vi "updateCVTCluster.vi"(1 "error in":errorcluster, 2 "variant (destination) out":variant, 3 "Cluster Names":string[](array[string]), 4 "CVT Names":string[](array[string])) -> (0 "error out":errorcluster)   [LabVIEW 2011]
uses:
  OnOffTypeDef.ctl
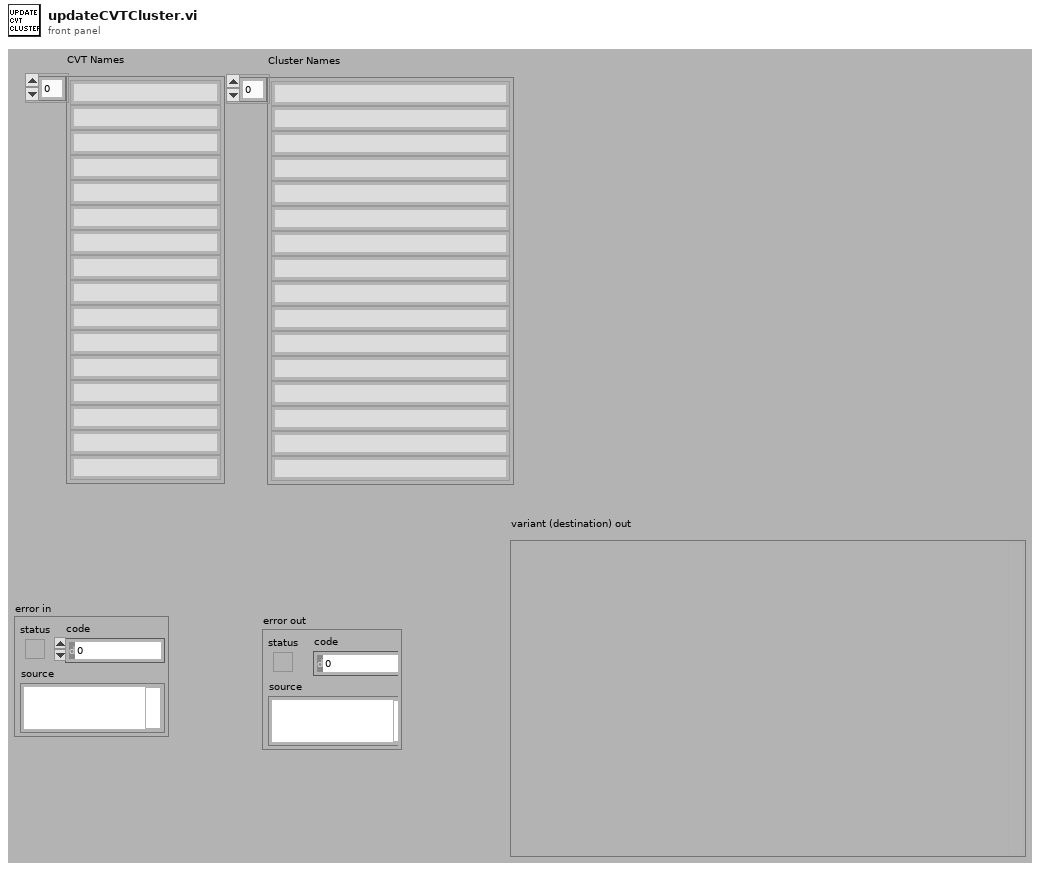
[diagram p1: front panel]
types:
  T1 = typedef "OnOffTypeDef.ctl" = enum16{"off", "on"}
  T2 = typedef "Type Descriptor Enumeration__ogtk.ctl" = enum8{"<Null>", "I8", "I16", "I32", "I64", "U8", "U16", "U32", "U64", "SGL", "DBL", "EXT", "CSG", "CDB", "CXT", "0x0F", "0x10", "0x11", "0x12", "0x13", "0x14", "Enum U8", "Enum U16", "Enum U32", "Enum U64", "SGL PQ", "DBL PQ", "EXT PQ", "CSG PQ", "CDB PQ", "CXT PQ", "0x1F", "0x20", "Boolean", "0x22", "0x23", "0x24", "0x25", "0x26", "0x27", "0x28", "0x29", "0x2A", "0x2B", "0x2C", "0x2D", "0x2E", "0x2F", "String", "0x31", "Path", "Pict", "0x34", "0x35", "0x36", "DAQ", "0x38", "0x39", "0x3A", "0x3B", "0x3C", "0x3D", "0x3E", "0x3F", "Array", "0x41", "0x42", "0x43", "0x44", "0x45", "0x46", "0x47", "0x48", "0x49", "0x4A", "0x4B", "0x4C", "0x4D", "0x4E", "0x4F", "Cluster", "0x51", "0x52", "Variant", "Waveform", "0x55", "0x56", "0x57", "0x58", "0x59", "0x5A", "0x5B", "0x5C", "0x5D", "0x5E", "0x5F", "0x60", "0x61", "0x62", "0x63", "0x64", "0x65", "0x66", "0x67", "0x68", "0x69", "0x6A", "0x6B", "0x6C", "0x6D", "0x6E", "0x6F", "Refnum"}
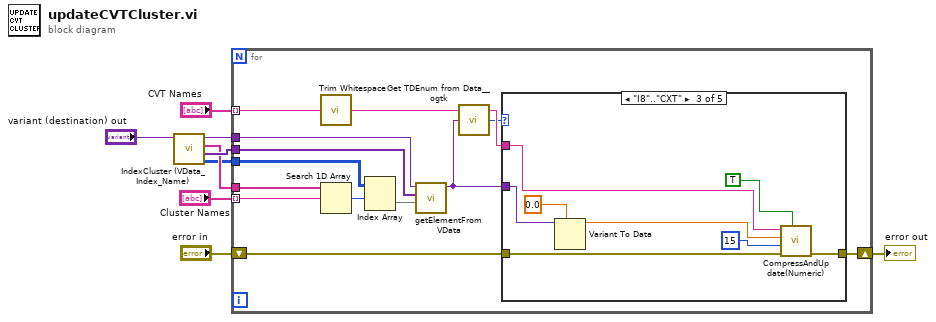
[diagram p0: block diagram]
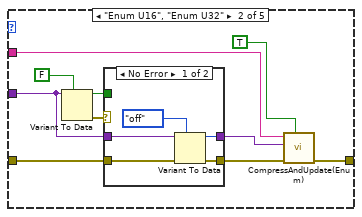
[diagram p3: hidden frame]
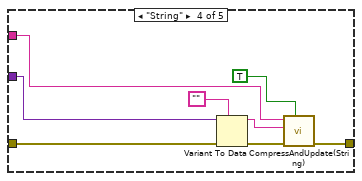
[diagram p5: hidden frame]
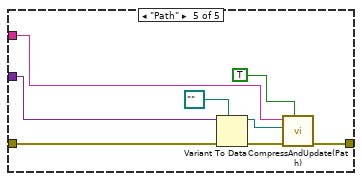
[diagram p6: hidden frame]
diagram:
  n1 = call "IndexCluster (VData_Index_Name).vi"("variant (destination)"="variant (destination) out") -> ("index Array"=w1:i32[][], "Array of VData"=w4:variant[], "Names (Array)"=w2:string[], "variant (destination)out"=w3:variant)  [unwired: 7 in]
  n2 = for {
    tunnel: "CVT Names" -> [w22] mode=indexing
    tunnel: "Cluster Names" -> [w14] mode=indexing
    shift-right: [w19] -> w6
    shift-left: "error in" -> [w20]
    tunnel: w4 -> [w17]
    tunnel: w3 -> [w16]
    tunnel: w2 -> [w15]
    tunnel: w1 -> [w13]
    n3 = call "Trim Whitespace.vi"("string"=w22) -> ("trimmed string"=w21:string)  [unwired: 1 in]
    n4 = Search 1D Array(1D array=w15, element=w14) -> (index of element=w12:i32)  [unwired: 1 in]
    n5 = Index Array(array=w13, index (row)=w12) -> (element=w11:i32[])  [unwired: 1 in]
    n6 = call "getElementFromVData.vi"("index Array 2"=w11, "Settings VData"=w17, "Cluster in"=w16) -> ("element out"=w10:variant)  [unwired: 7 in, 1 out]
    n7 = call "Get TDEnum from Data__ogtk.vi"("Data"=w10) -> ("Type Descriptor Enumeration"=w18:T2)  [unwired: 4 in]
    n8 = case shown="\"I8\"..\"CXT\"" w18 {
      tunnel: w10 -> [_ w31 w43 w54 w62]
      tunnel: w21 -> [_ w30 w46 w55 w63]
      tunnel: [w23 w27 w44 w51 w61] -> w19
      tunnel: w20 -> [w23 w25 w42 w50 w60]
      frame "<Null>", Default {
      }
      frame "Enum U16", "Enum U32" {
        n9 = Variant To Data(type=FALSE, Variant=w31) -> (data=w32:bool, error out=w33:errorcluster)  [unwired: 1 in]
        n10 = case shown="No Error" w33 {
          tunnel: w32 -> [_ _]
          tunnel: [w36 w40] -> w29
          tunnel: w31 -> [w38 w40]
          tunnel: w25 -> [w35 w39]
          tunnel: [w34 w39] -> w24
          frame No Error {
            n11 = Variant To Data(error in=w35, type=OnOffTypeDef."off" ("Save"), Variant=w38) -> (data=w36:T1, error out=w34:errorcluster)
          }
          frame Error {
          }
        }
        n12 = call "CompressAndUpdate(Enum).vi"("force CVT update (false)"=TRUE, "error in"=w24, "enum variant"=w29, "command or variable name"=w30) -> ("error out"=w27:errorcluster)  [unwired: 7 in]
      }
      frame "I8".."CXT" {
        n13 = Variant To Data(type=0.0, Variant=w43) -> (data=w47:dbl)  [unwired: 1 in, 1 out]
        n14 = call "CompressAndUpdate(Numeric).vi"("force CVT update (false)"=TRUE, "error in"=w42, "precision (6)"=i16 15, "Numeric"=w47, "command or variable name"=w46) -> ("error out"=w44:errorcluster)  [unwired: 6 in]
      }
      frame "String" {
        n15 = Variant To Data(error in=w50, type="", Variant=w54) -> (data=w52:string, error out=w49:errorcluster)
        n16 = call "CompressAndUpdate(String).vi"("force CVT update (false)"=TRUE, "error in"=w49, "String"=w52, "command or variable name"=w55) -> ("error out"=w51:errorcluster)  [unwired: 7 in]
      }
      frame "Path" {
        n17 = Variant To Data(error in=w60, type=path "", Variant=w62) -> (data=w57:path, error out=w59:errorcluster)
        n18 = call "CompressAndUpdate(Path).vi"("force CVT update (false)"=TRUE, "error in"=w59, "Path"=w57, "command or variable name"=w63) -> ("error out"=w61:errorcluster)  [unwired: 7 in]
      }
    }
  }
  "error out" <- w6
